vi "Path_Check if File or Folder Exists.vi"(11 "File or Folder Path in":path) -> (2 "File or Folder Found?":bool, 3 "File or Folder Path dub":path)   [LabVIEW 2020, in "ClassLoader.lvlib"]
uses:
  ClassLoader.lvlib
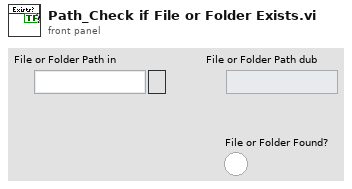
[diagram p1: front panel]
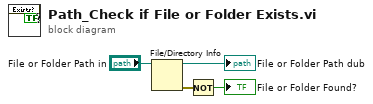
[diagram p0: block diagram]
diagram:
  n1 = File/Directory Info(path="File or Folder Path in") -> (path out=→"File or Folder Path dub":path, error out=w2:errorcluster)  [unwired: 1 in, 5 out]
  n2 = Not(x=w2) -> (.not. x?=→"File or Folder Found?":bool)
